vi "Initialize.vi"(8 "error in":errorcluster, 9 "Application Directory":path, 10 "Device":string="Report", 11 "Report in":refnum<class "Report.lvclass">) -> (0 "error out":errorcluster, 3 "Report out":refnum<class "Report.lvclass">)   [LabVIEW 2023, in "Report.lvlib" / "Report.lvclass"]
uses:
  Report.lvclass
  C:/Users/Public/Documents/Development/builds/Engine/Engine.lvlibp/Project/Engine.lvclass
  builds/Engine/Engine.lvlibp/Accessors/Read Directory.vi
  builds/Tools/Config.lvlibp/Config.lvclass
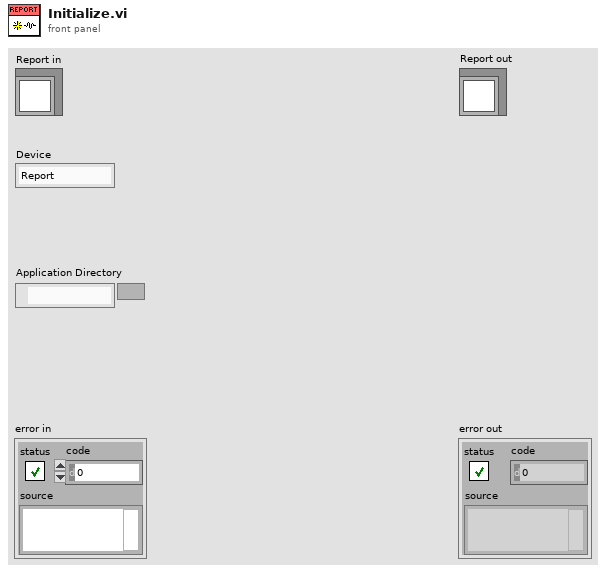
[diagram p1: front panel]
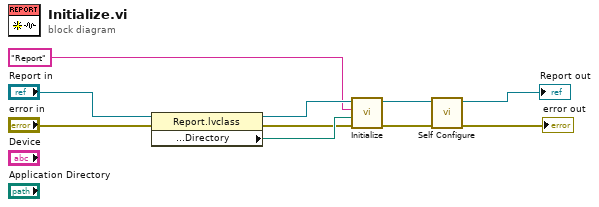
[diagram p0: block diagram]
diagram:
  n1 = property class="Report.lvclass"(reference="Report in", error in="error in") -> (reference out=w6:refnum<class "Report.lvclass">, error out=w1:errorcluster, "Accessors:Application:Information:Directory"=w5:path)
  n2 = call-parent "Initialize.vi"("error in"=w1, "Path"=w5, "Device"="Report" ("Device \n(Case Sensitive)"), "Config in"=w6) -> ("error out"=w3:errorcluster, "Config out"=w8:refnum<class "Report.lvclass">)  [unwired: 6 in]
  n3 = call "Self Configure.vi"("error in"=w3, "Report in"=w8) -> ("error out"=→"error out":errorcluster, "Report out"=→"Report out":refnum<class "Report.lvclass">)  [unwired: 8 in]
